vi "ServoPosReadIn.vi"(10 "Command":string="UU\u0001\u0005\u001cþÿà") -> (1 "Angel":dbl min=0.0 max=240.0 step=0.24, 2 "ID":u8=1)   [LabVIEW 2013]
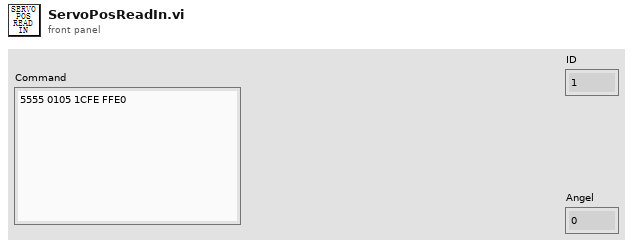
[diagram p1: front panel]
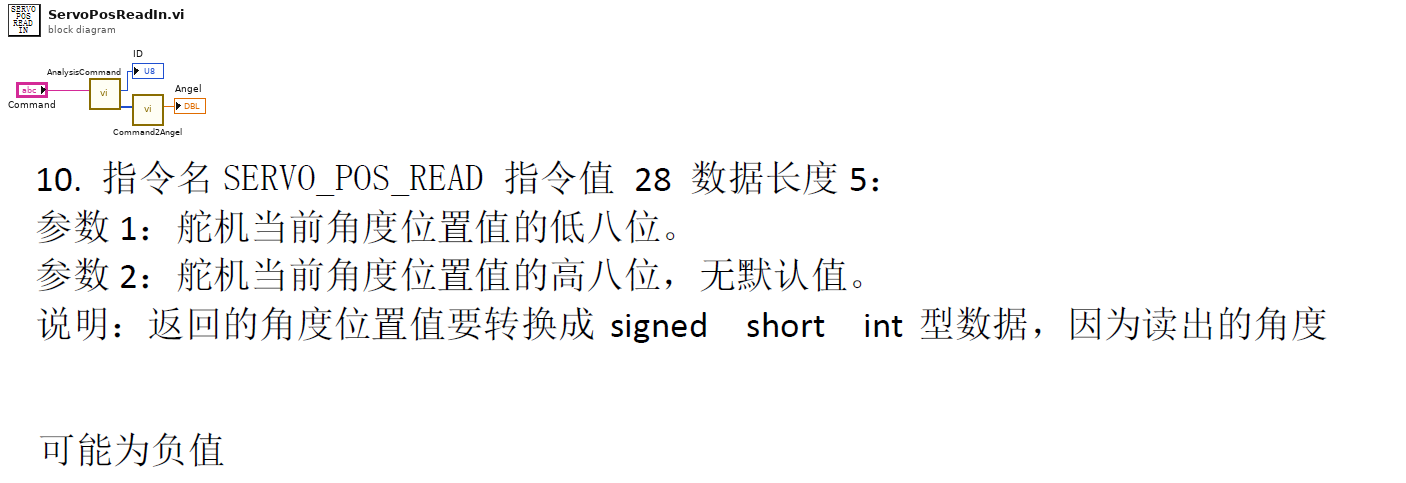
[diagram p0: block diagram]
diagram:
  n1 = call "AnalysisCommand.vi"("Command"="Command") -> ("DataOut"=w2:u8[], "ID"=→"ID":u8)  [unwired: 8 in, 1 out]
  n2 = call "Command2Angel.vi"("DataIn"=w2) -> ("AngelOut"=→"Angel":dbl)  [unwired: 10 in]
